vi "scaleFactor.set.vi"(8 "error in (no error)":errorcluster, 10 "scaleFactor":dbl, 11 "scaleFactor in":refnum<class "scaleFactor.lvclass">) -> (0 "error out":errorcluster, 3 "scaleFactor out":refnum<class "scaleFactor.lvclass">)   [LabVIEW 2020, in "nominal types.lvlib" / "timestampManifest.lvlib" / "scaleFactor.lvclass"]
uses:
  scaleFactor.lvclass
  scaleFactor.lvclass/scaleFactor.ctl
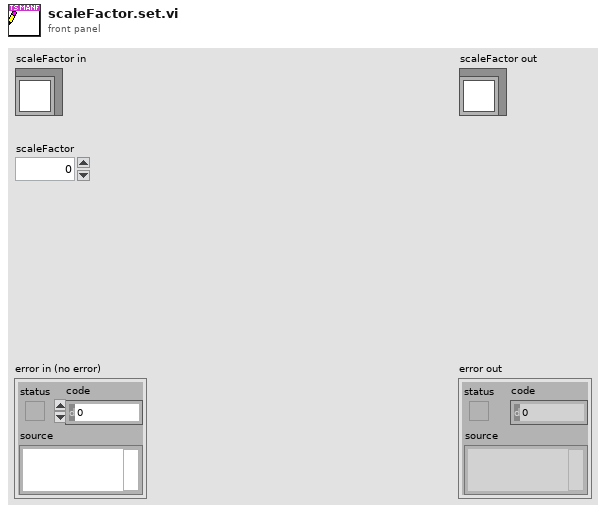
[diagram p1: front panel]
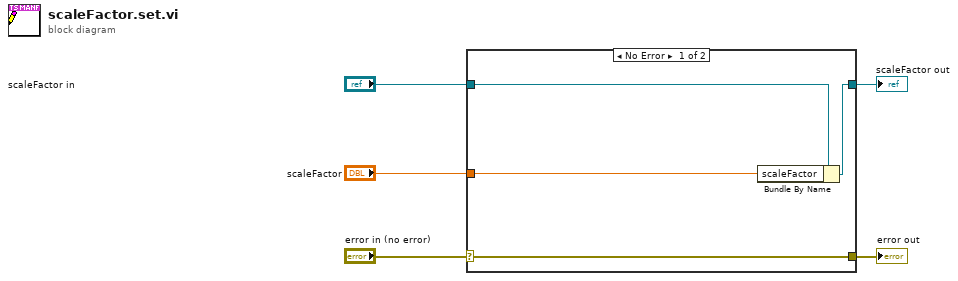
[diagram p0: block diagram]
diagram:
  n1 = case shown="No Error" "error in (no error)" {
    selector: "error in (no error)" -> [w9 w10]
    tunnel: [w9 w10] -> w4
    tunnel: [w7 w11] -> w2
    tunnel: "scaleFactor in" -> [w8 w11]
    tunnel: "scaleFactor" -> [w6 _]
    frame No Error {
      n2 = Bundle By Name(cluster=w8, "scaleFactor"=w6) -> (w7:refnum<class "scaleFactor.lvclass">)
    }
    frame Error {
    }
  }
  "error out" <- w4
  "scaleFactor out" <- w2
